vi "midi-track.get_song_length.vi"(8 "error in (no error)":errorcluster, 11 "midi-file-events in":refnum<class "midi-file-events.lvclass">) -> (0 "error out":errorcluster, 2 "Song Length (s)":dbl, 3 "midi-file-events out":refnum<class "midi-file-events.lvclass">)   [LabVIEW 2020, in "midi-file-events.lvclass"]
uses:
  midi-file-events.lvclass
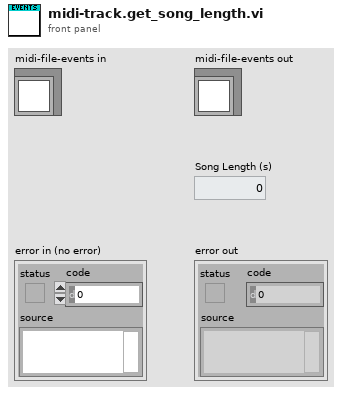
[diagram p1: front panel]
types:
  T1 = map{dbl, set{refnum<class "midi-file-event.midi.lvclass">}}
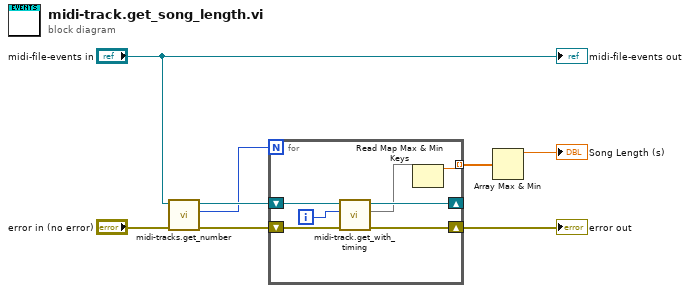
[diagram p0: block diagram]
diagram:
  n1 = call "midi-tracks.get_number.vi"("error in (no error)"="error in (no error)", "midi-file-events in"="midi-file-events in") -> ("error out"=w5:errorcluster, "Numer of Tracks"=w7:i32, "midi-file-events out"=w8:refnum<class "midi-file-events.lvclass">)  [unwired: 7 in]
  n2 = for {
    N: w7 -> [_]
    shift-right: [w13] -> _
    shift-left: w8 -> [w15]
    tunnel: [w11] -> w6 mode=indexing
    shift-right: [w9] -> w3
    shift-left: w5 -> [w10]
    i -> [w14]
    n3 = call "midi-track.get_with_timing.vi"("error in (no error)"=w10, "Track Number"=w14, "midi-file-events in"=w15) -> ("error out"=w9:errorcluster, "Events by time"=w12:T1, "midi-file-events out"=w13:refnum<class "midi-file-events.lvclass">)  [unwired: 6 in]
    n4 = Read Map Max & Min Keys(11:w12) -> (3:w11:dbl)  [unwired: 1 out]
  }
  "error out" <- w3
  n5 = Array Max & Min(array=w6) -> (max value=→"Song Length (s)":dbl)  [unwired: 3 out]
  "midi-file-events out" <- "midi-file-events in"
